vi "blockStats.vi"() -> ()   [LabVIEW 2013]
uses:
  Controls/blocksPP.ctl
  <vilib>/Analysis/baseanly.llb/Mean (DBL).vi
  Globals/measurementGlobal.vi
  <vilib>/Analysis/NI_AALBase.lvlib
panel:
  out "appended array":dbl[](array[numeric])
  out "Numeric":i32
  out "output array":T1[](array[typedef])
  out "moment":dbl format="%0.2f"
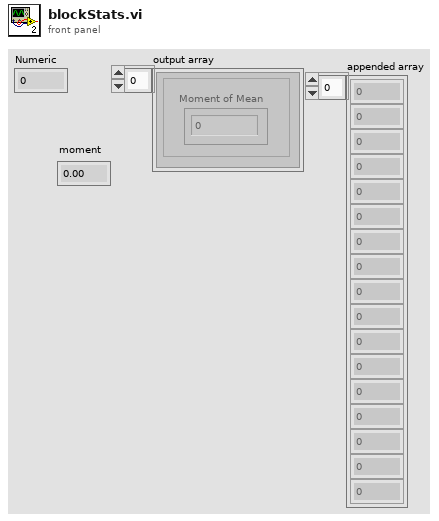
[diagram p1: front panel]
types:
  T1 = typedef "blocksPP.ctl" = cluster{"Moment of Mean":dbl}
  T2 = typedef "postProData.ctl" = cluster{"Channel":string, "Samples":i32, "Mean":dbl, "Standard Deviation":dbl}
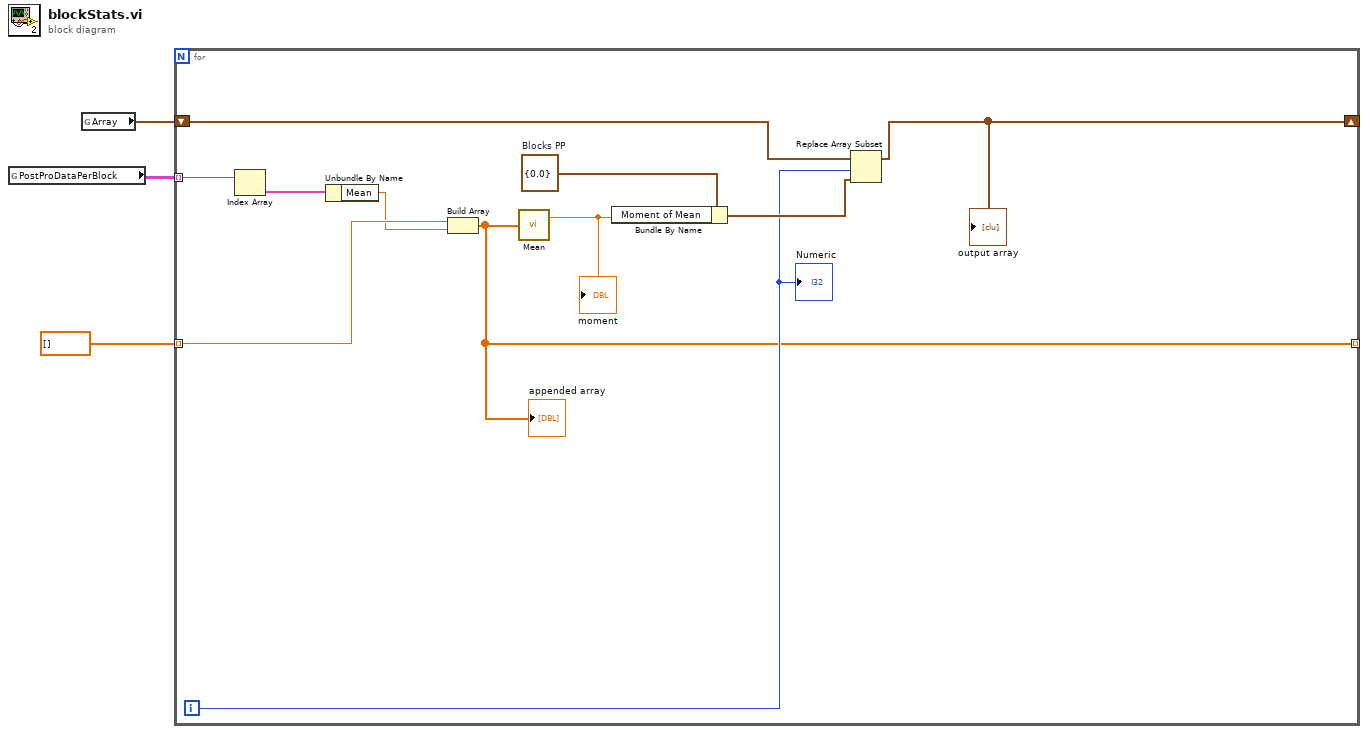
[diagram p0: block diagram]
diagram:
  n1 = global read "measurementGlobal.vi" "PostProDataPerBlock"() -> (w3:T2[][])
  n2 = global read "measurementGlobal.vi" "Array"() -> (w1:T1[])
  n3 = for {
    tunnel: w3 -> [w14] mode=indexing
    shift-right: [w7] -> _
    shift-left: w1 -> [w10]
    tunnel: dbl[] [] -> [w12] mode=indexing
    tunnel: [w4] -> _ mode=indexing
    i -> [w8]
    w11 = T1 {"Moment of Mean"=0.0}  # Blocks PP
    n4 = Index Array(array=w14) -> (element=w13:T2)  [unwired: 1 in]
    n5 = Unbundle By Name(w13) -> ("Mean"=w6:dbl)
    n6 = Build Array(w12, w6) -> (w4:dbl[])
    "appended array" <- w4
    n7 = call-poly <vilib>:"Mean.vi"("X"=w4) -> ("mean"=w5:dbl)  [unwired: 1 out]
    "moment" <- w5
    n8 = Bundle By Name(cluster=w11, "Moment of Mean"=w5) -> (w9:T1)
    n9 = Replace Array Subset(array=w10, new element=w9, index=w8) -> (w7:T1[])
    "output array" <- w7
    "Numeric" <- w8
  }
